vi "Traction Control.vi"(11 "stop":bool) -> ()   [LabVIEW 2015]
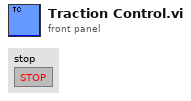
[diagram p1: front panel]
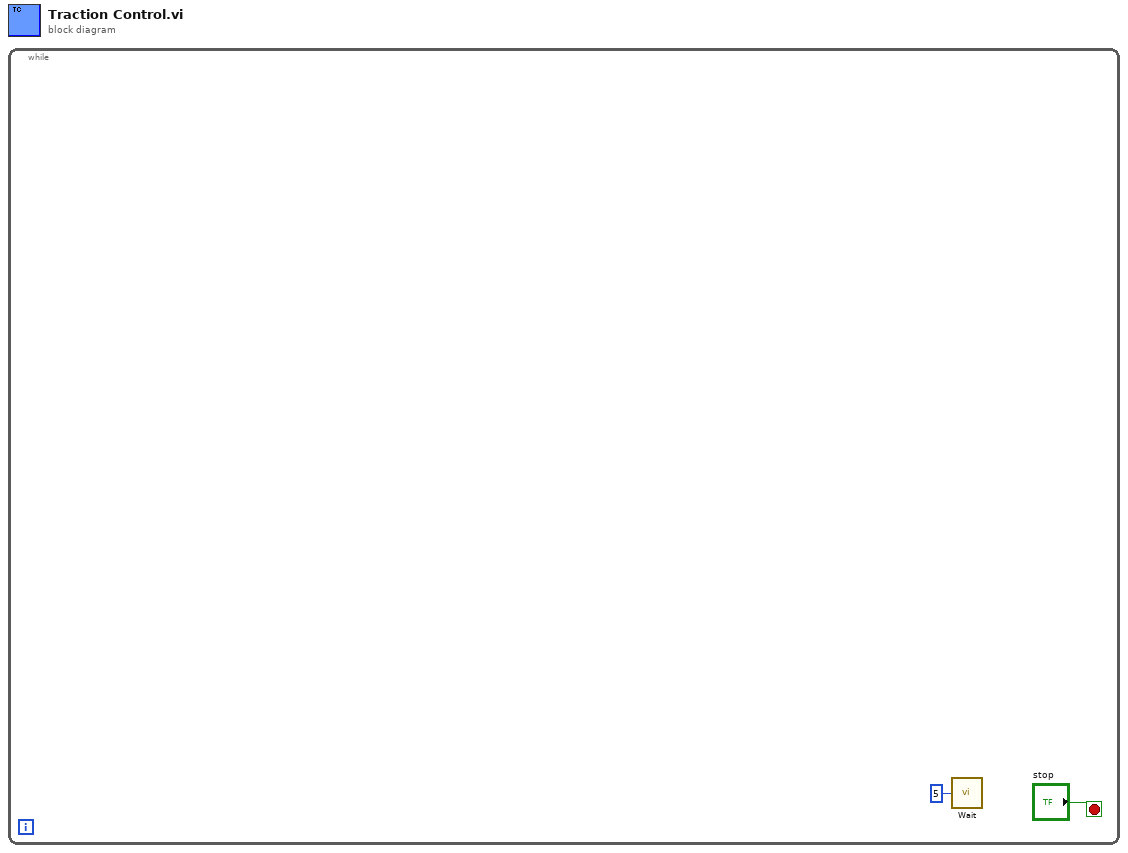
[diagram p0: block diagram]
diagram:
  n1 = while {
    stop <- "stop" stop-if-true
    n2 = call "Wait"("Count(mSec)"=u32 5) -> ()  [unwired: 1 out]
  }
